vi "ABB Load-Save config.vi"(10 "confirm save":bool, 11 "Mode":enum16{"LOAD", "SAVE"}(ring)) -> ()   [LabVIEW 2017]
uses:
  ABB global.vi
panel:
  out "first row":string[](array[string])
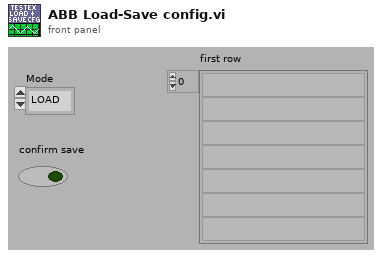
[diagram p1: front panel]
types:
  T1 = cluster{"First row[0]":string, "First row[1]":string, "First row[2]":string, "First row[3]":string, "First row[4]":string}
  T2 = cluster{"First row[0]":string, "First row[1]":string, "First row[2]":string, "First row[3]":string, "First row[4]":string, "First row[5]":string, "First row[6]":string, "First row[7]":string, "First row[8]":string}
  T3 = cluster{"Number Values":i32, "Tolerance":dbl, "Value (ratio) ":dbl[], "Hold time (sec)":dbl}
  T4 = cluster{"Thermal Stability (deg/hr)":dbl, "Reading interval (mins)":dbl}
  T5 = cluster{"Number Values":i32, "Tolerance ":dbl, "Value (ratio)":dbl[], "Hold time (sec)":dbl}
  T6 = cluster{"Simulate Norma":bool, "Norma 5000 Address":u8, "WebDaq IP Address":string, "Simulate cDAQ":bool}
  T7 = cluster{"temp. alloc":i32[], "category":i32[], "Category names":string[], "Category none names":string[]}
  T8 = cluster{"Number of Loads":i32, "Loads (%Rated)":dbl[]}
  T9 = cluster{"VT Primary":dbl, "VT Secondary":dbl, "CT  Primary":dbl, "CT Secondary":dbl, "Current Shunt":enum16{"Internal", "External"}, "Averaging interval":dbl}
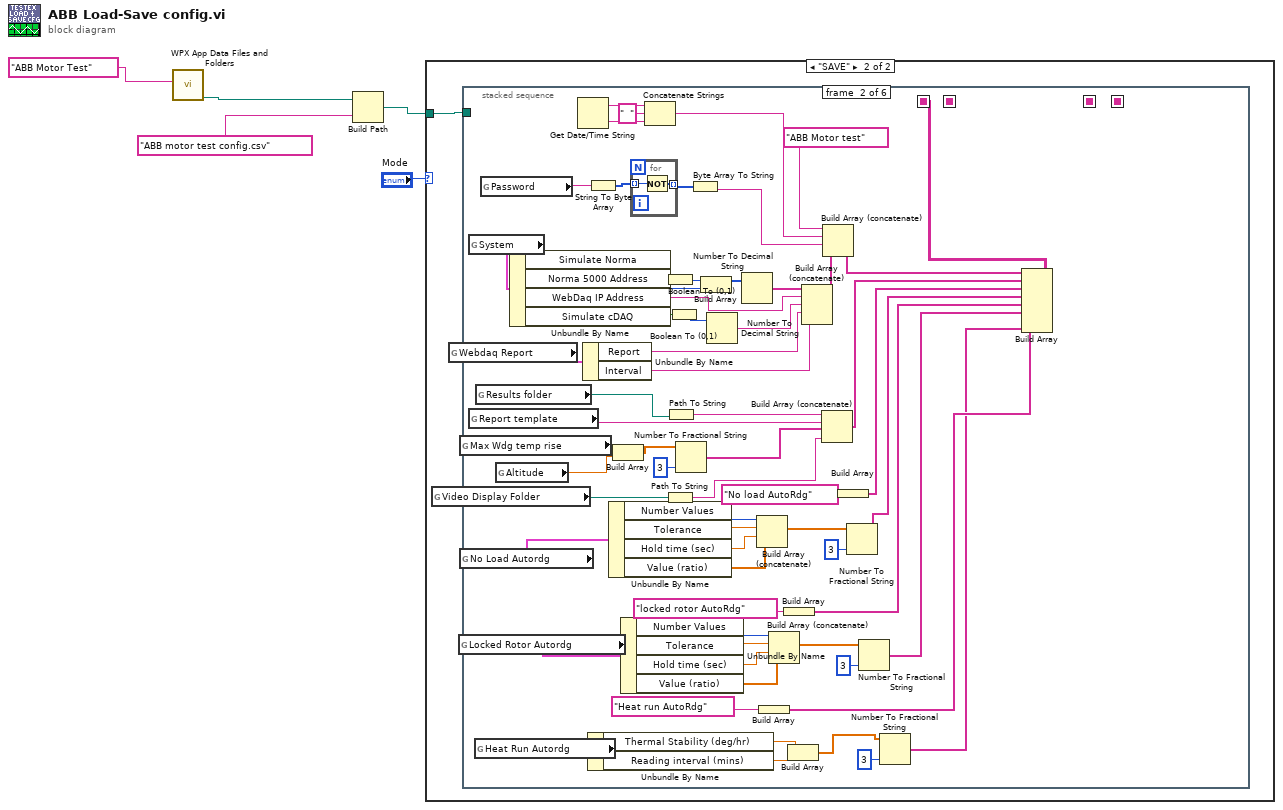
[diagram p0: block diagram]
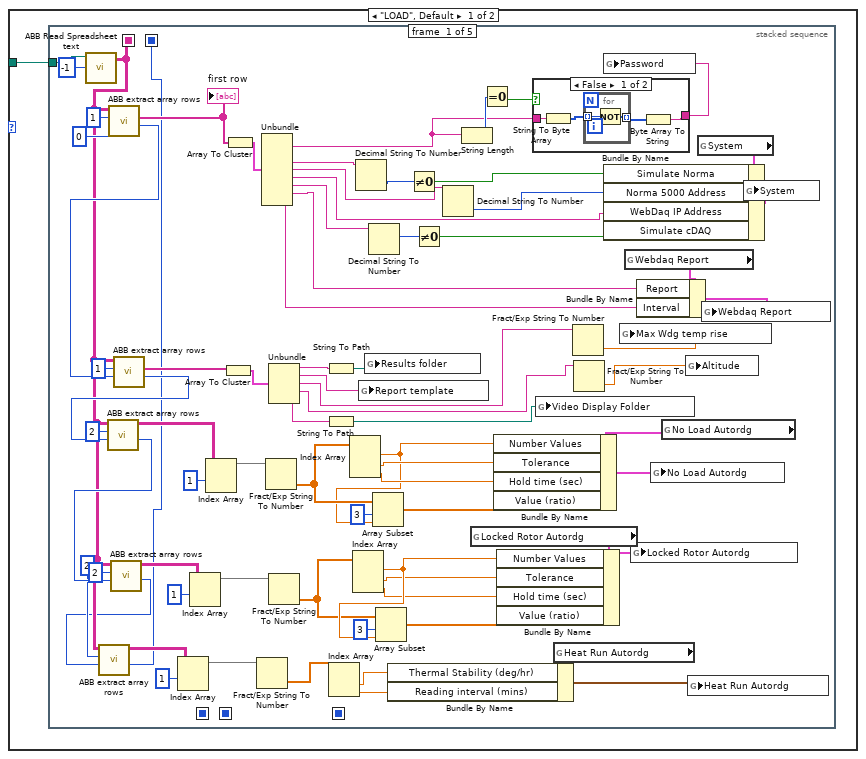
[diagram p2: hidden frame]
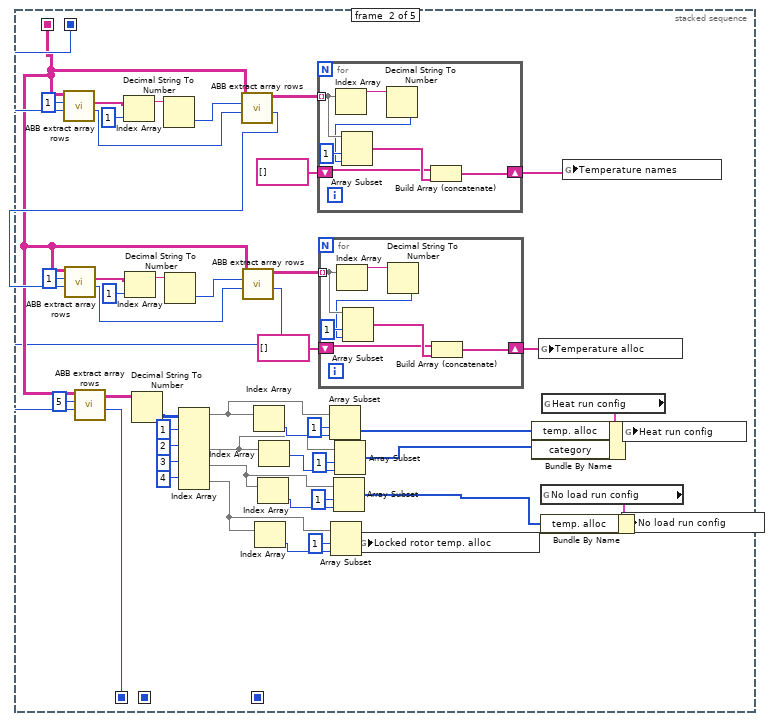
[diagram p4: hidden frame]
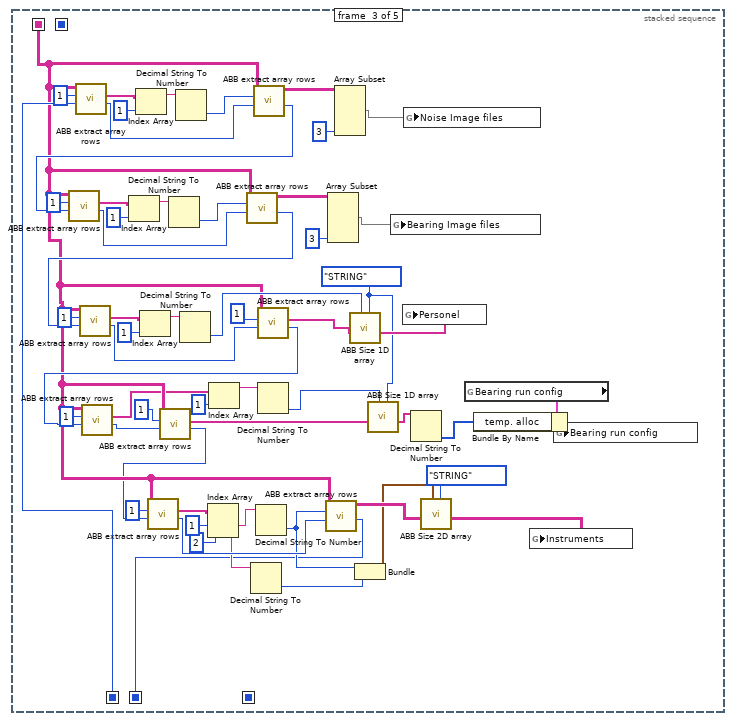
[diagram p5: hidden frame]
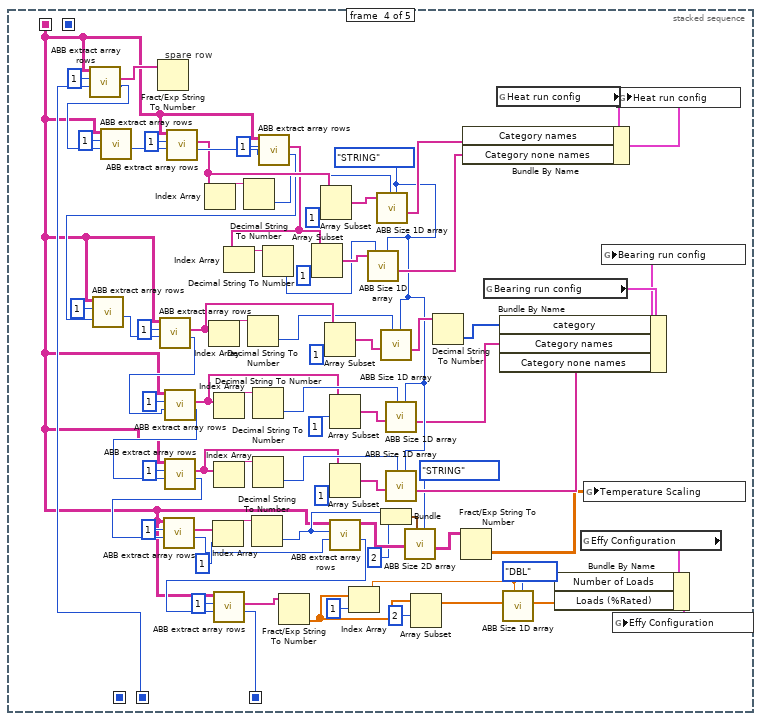
[diagram p6: hidden frame]
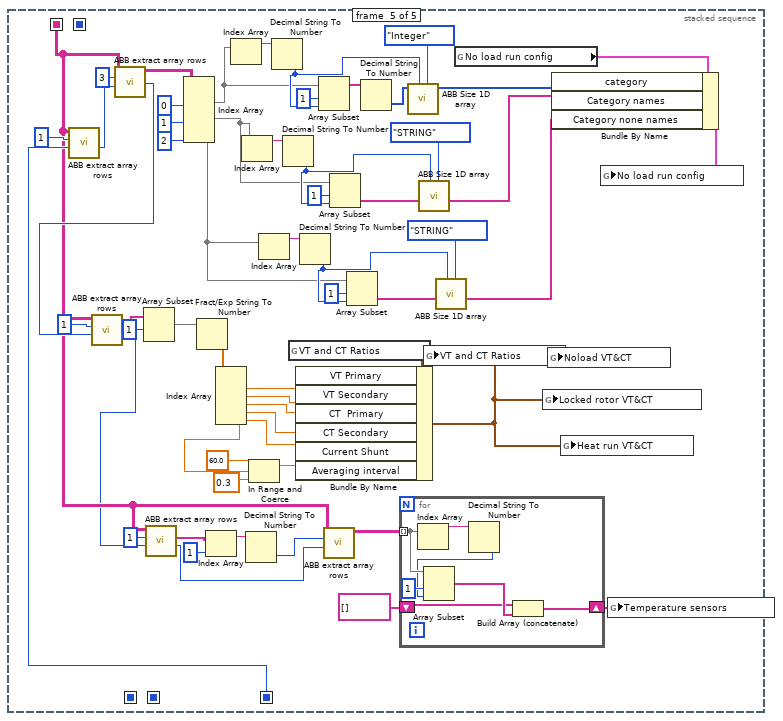
[diagram p7: hidden frame]
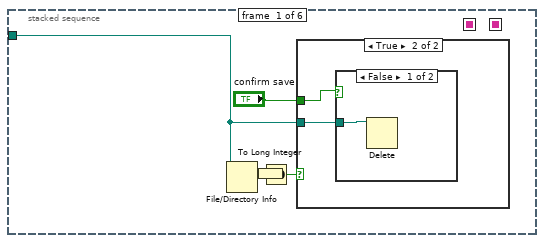
[diagram p8: hidden frame]
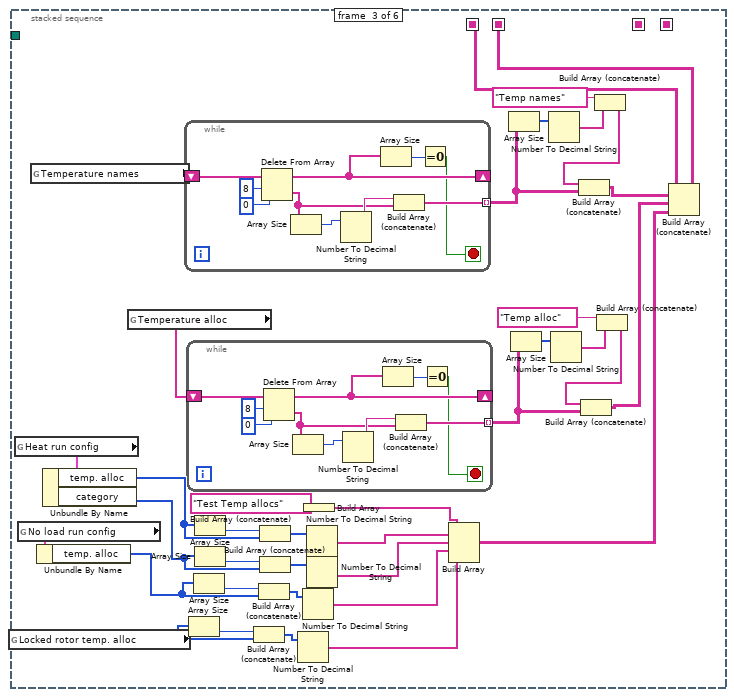
[diagram p11: hidden frame]
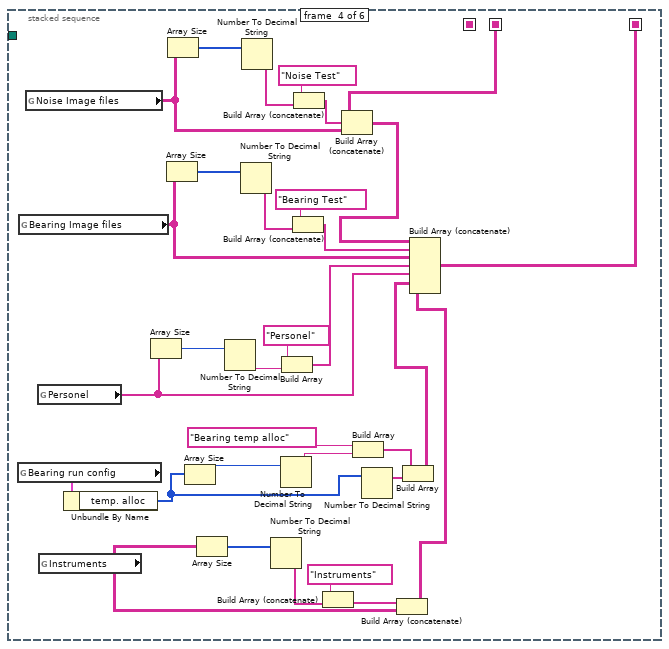
[diagram p12: hidden frame]
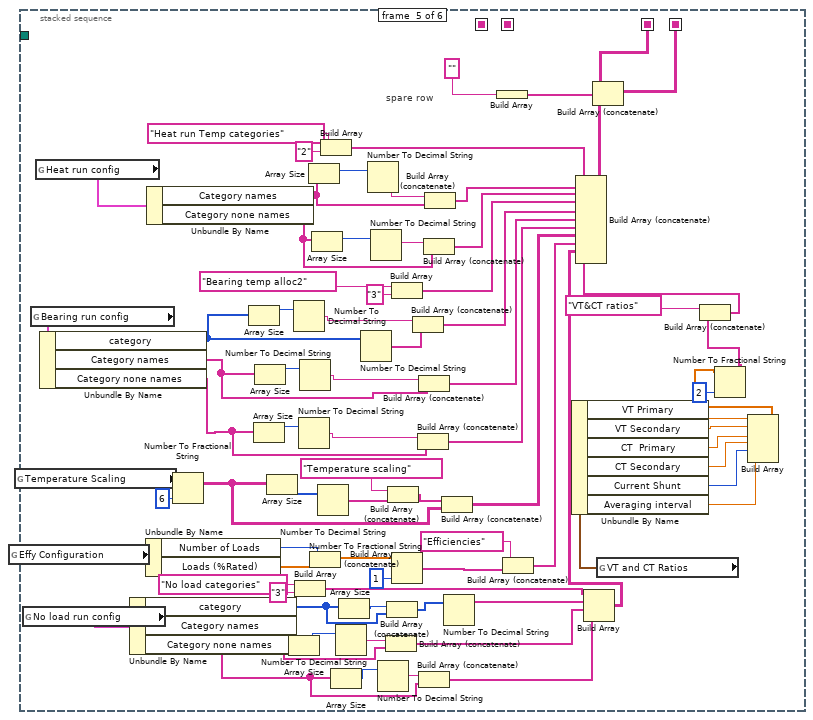
[diagram p13: hidden frame]
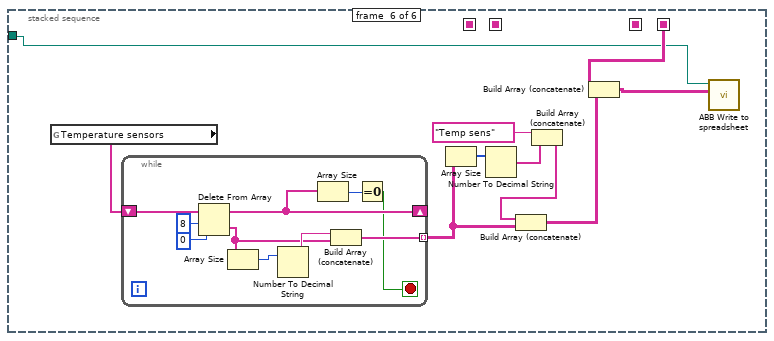
[diagram p14: hidden frame]
diagram:
  n1 = call "WPX App Data Files and Folders.vi"("ApplicationName"="ABB Motor Test") -> ("DataFolder"=w1:path)  [unwired: 7 in, 3 out]
  n2 = Build Path(base path=w1, name or relative path="ABB motor test config.csv") -> (appended path=w3:path)
  n3 = case shown="\"SAVE\"" "Mode" {
    tunnel: w3 -> [w6 w360]
    frame "LOAD", Default {
      n4 = stacked-sequence {
        seq-local: [w30 _ _ _ _] -> [_ w118 w162 w215 w295]
        seq-local: [w23 _ _ _ _] -> [_ w138 _ _ _]
        seq-local: [_ w103 _ _ _] -> [_ _ w207 _ _]
        seq-local: [_ _ w166 _ _] -> [_ _ _ w292 _]
        seq-local: [_ _ _ w214 _] -> [_ _ _ _ w351]
        tunnel: w6 -> [w77 _ _ _ _]
        frame #0 {
          n5 = call "ABB Read Spreadsheet text.vi"("number of rows (all:-1)"=-1, "file path (dialog if empty)"=w77) -> ("all rows"=w30:string[][])  [unwired: 5 in, 4 out]
          n6 = call "ABB extract array rows.vi"("Row offset"=0, "# rows"=1, "Input array"=w30) -> ("Next row"=w65:i32, "First row"=w74:string[])  [unwired: 6 in, 1 out]
          "first row" <- w74
          n7 = call "ABB extract array rows.vi"("Row offset"=w65, "# rows"=1, "Input array"=w30) -> ("Next row"=w59:i32, "First row"=w64:string[])  [unwired: 6 in, 1 out]
          n8 = call "ABB extract array rows.vi"("Row offset"=w59, "# rows"=2, "Input array"=w30) -> ("Next row"=w35:i32, "All rows"=w58:string[][])  [unwired: 6 in, 1 out]
          n9 = call "ABB extract array rows.vi"("Row offset"=w35, "# rows"=2, "Input array"=w30) -> ("Next row"=w29:i32, "All rows"=w37:string[][])  [unwired: 6 in, 1 out]
          n10 = call "ABB extract array rows.vi"("Row offset"=w29, "# rows"=2, "Input array"=w30) -> ("Next row"=w23:i32, "All rows"=w33:string[][])  [unwired: 6 in, 1 out]
          n11 = Index Array(array=w33, index (row)=1) -> (element=w31:string[])  [unwired: 1 in]
          n12 = Index Array(array=w37, index (row)=1) -> (element=w39:string[])  [unwired: 1 in]
          n13 = Index Array(array=w58, index (row)=1) -> (element=w56:string[])  [unwired: 1 in]
          n14 = Array To Cluster(array=w64) -> (cluster=w63:T1)
          n15 = Array To Cluster(array=w74) -> (cluster=w82:T2)
          n16 = Fract/Exp String To Number(string=w31) -> (number=w27:dbl[])  [unwired: 3 in, 1 out]
          n17 = Unbundle(w82) -> ("First row[2]"=w76:string, "First row[3]"=w72:string, "First row[4]"=w21:string, "First row[5]"=w20:string, "First row[6]"=w19:string, "First row[7]"=w9:string, "First row[8]"=w10:string)  [unwired: 2 out]
          n18 = Fract/Exp String To Number(string=w56) -> (number=w52:dbl[])  [unwired: 3 in, 1 out]
          n19 = Unbundle(w63) -> ("First row[0]"=w62:string, "First row[1]"=w22:string, "First row[2]"=w16:string, "First row[3]"=w15:string, "First row[4]"=w8:string)
          n20 = Fract/Exp String To Number(string=w39) -> (number=w43:dbl[])  [unwired: 3 in, 1 out]
          n21 = String To Path(string=w62) -> (path=w61:path)
          n22 = String To Path(string=w8) -> (path=w7:path)
          n23 = Index Array(array=w27) -> (element #1=w26:dbl, element #2=w25:dbl)  [unwired: 2 in]
          n24 = Index Array(array=w52) -> (element #1=w50:dbl, element #2=w54:dbl, element #3=w53:dbl)  [unwired: 3 in]
          n25 = Index Array(array=w43) -> (element #1=w45:dbl, element #2=w41:dbl, element #3=w42:dbl)  [unwired: 3 in]
          n26 = Decimal String To Number(string=w72) -> (number=w71:i32)  [unwired: 2 in, 1 out]
          n27 = global write "ABB global.vi" "Report template"(w22) -> ()
          n28 = global write "ABB global.vi" "Results folder"(w61) -> ()
          n29 = Decimal String To Number(string=w19) -> (number=w18:i32)  [unwired: 2 in, 1 out]
          n30 = Array Subset(array=w52, index=3, length=w50) -> (w49:dbl[])
          n31 = Array Subset(array=w43, index=3, length=w45) -> (w46:dbl[])
          n32 = Not Equal To 0?(x=w71) -> (x != 0?=w69:bool)
          n33 = Not Equal To 0?(x=w18) -> (x != 0?=w17:bool)
          n34 = Decimal String To Number(string=w21) -> (number=w68:i32)  [unwired: 2 in, 1 out]
          n35 = String Length(string=w76) -> (length=w81:i32)
          n36 = global read "ABB global.vi" "Locked Rotor Autordg"() -> (w40:T3)
          n37 = Equal To 0?(x=w81) -> (x = 0?=w80:bool)
          n38 = Bundle By Name(cluster=w40, "Number Values"=w45, "Tolerance"=w41, "Hold time (sec)"=w42, "Value (ratio)"=w46) -> (w47:T3)
          n39 = case shown="False" w80 {
            tunnel: w76 -> [w84 w89]
            tunnel: [w83 w89] -> w79
            frame False {
              n40 = String To Byte Array(string=w84) -> (unsigned byte array=w86:u8[])
              n41 = for {
                tunnel: w86 -> [w88] mode=indexing
                tunnel: [w87] -> w85 mode=indexing
                n42 = Not(x=w88) -> (.not. x?=w87:u8)
              }
              n43 = Byte Array To String(unsigned byte array=w85) -> (string=w83:string)
            }
            frame True {
            }
          }
          n44 = global write "ABB global.vi" "Video Display Folder"(w7) -> ()
          n45 = global read "ABB global.vi" "Heat Run Autordg"() -> (w28:T4)
          n46 = Bundle By Name(cluster=w28, "Thermal Stability (deg/hr)"=w26, "Reading interval (mins)"=w25) -> (w24:T4)
          n47 = Fract/Exp String To Number(string=w16) -> (number=w14:dbl)  [unwired: 3 in, 1 out]
          n48 = Fract/Exp String To Number(string=w15) -> (number=w13:dbl)  [unwired: 3 in, 1 out]
          n49 = global write "ABB global.vi" "Password"(w79) -> ()
          n50 = global write "ABB global.vi" "Max Wdg temp rise"(w14) -> ()
          n51 = global read "ABB global.vi" "Webdaq Report"() -> (w12:cluster{"Report":string, "Interval":string})
          n52 = global write "ABB global.vi" "Locked Rotor Autordg"(w47) -> ()
          n53 = Bundle By Name(cluster=w12, "Report"=w9, "Interval"=w10) -> (w11:cluster{"Report":string, "Interval":string})
          n54 = global read "ABB global.vi" "No Load Autordg"() -> (w55:T5)
          n55 = Bundle By Name(cluster=w55, "Number Values"=w50, "Tolerance"=w54, "Hold time (sec)"=w53, "Value (ratio)"=w49) -> (w48:T5)
          n56 = global write "ABB global.vi" "No Load Autordg"(w48) -> ()
          n57 = global write "ABB global.vi" "Altitude"(w13) -> ()
          n58 = global write "ABB global.vi" "Heat Run Autordg"(w24) -> ()
          n59 = global read "ABB global.vi" "System"() -> (w70:T6)
          n60 = Bundle By Name(cluster=w70, "Simulate Norma"=w69, "Norma 5000 Address"=w68, "WebDaq IP Address"=w20, "Simulate cDAQ"=w17) -> (w67:T6)
          n61 = global write "ABB global.vi" "Webdaq Report"(w11) -> ()
          n62 = global write "ABB global.vi" "System"(w67) -> ()
        }
        frame #1 {
          n63 = call "ABB extract array rows.vi"("Row offset"=w138, "# rows"=1, "Input array"=w118) -> ("Next row"=w134:i32, "First row"=w137:string[])  [unwired: 6 in, 1 out]
          n64 = Index Array(array=w137, index=1) -> (element=w135:string)
          n65 = Decimal String To Number(string=w135) -> (number=w133:i32)  [unwired: 2 in, 1 out]
          n66 = call "ABB extract array rows.vi"("Row offset"=w134, "# rows"=w133, "Input array"=w118) -> ("Next row"=w121:i32, "All rows"=w132:string[][])  [unwired: 6 in, 1 out]
          n67 = call "ABB extract array rows.vi"("Row offset"=w121, "# rows"=1, "Input array"=w118) -> ("Next row"=w126:i32, "First row"=w123:string[])  [unwired: 6 in, 1 out]
          n68 = Index Array(array=w123, index=1) -> (element=w125:string)
          n69 = Decimal String To Number(string=w125) -> (number=w127:i32)  [unwired: 2 in, 1 out]
          n70 = call "ABB extract array rows.vi"("Row offset"=w126, "# rows"=w127, "Input array"=w118) -> ("Next row"=w112:i32, "All rows"=w128:string[][])  [unwired: 6 in, 1 out]
          n71 = call "ABB extract array rows.vi"("Row offset"=w112, "# rows"=5, "Input array"=w118) -> ("Next row"=w103:i32, "All rows"=w117:string[][])  [unwired: 6 in, 1 out]
          n72 = Decimal String To Number(string=w117) -> (number=w116:i32[][])  [unwired: 2 in, 1 out]
          n73 = Index Array(array=w116, index (row) #1=1 ("index (row)"), index (row) #2=2 ("index (row)"), index (row) #3=3 ("index (row)"), index (row) #4=4 ("index (row)")) -> (element #1=w110:i32[], element #2=w97:i32[], element #3=w95:i32[], element #4=w94:i32[])  [unwired: 4 in]
          n74 = Index Array(array=w110) -> (element=w111:i32)  [unwired: 1 in]
          n75 = Index Array(array=w94) -> (element=w106:i32)  [unwired: 1 in]
          n76 = Index Array(array=w95) -> (element=w107:i32)  [unwired: 1 in]
          n77 = Index Array(array=w97) -> (element=w93:i32)  [unwired: 1 in]
          n78 = for {
            tunnel: w132 -> [w153] mode=indexing
            shift-right: [w147] -> w130
            shift-left: string[] [] -> [w148]
            n79 = Index Array(array=w153) -> (element=w151:string)  [unwired: 1 in]
            n80 = Decimal String To Number(string=w151) -> (number=w150:i32)  [unwired: 2 in, 1 out]
            n81 = Array Subset(array=w153, index=1, length=w150) -> (w149:string[])
            n82 = Build Array (concatenate)(w148, w149) -> (w147:string[])
          }
          n83 = for {
            tunnel: w128 -> [w146] mode=indexing
            shift-right: [w140] -> w120
            shift-left: string[] [] -> [w141]
            n84 = Index Array(array=w146) -> (element=w144:string)  [unwired: 1 in]
            n85 = Decimal String To Number(string=w144) -> (number=w143:i32)  [unwired: 2 in, 1 out]
            n86 = Array Subset(array=w146, index=1, length=w143) -> (w142:string[])
            n87 = Build Array (concatenate)(w141, w142) -> (w140:string[])
          }
          n88 = Array Subset(array=w110, index=1, length=w111) -> (w100:i32[])
          n89 = Array Subset(array=w94, index=1, length=w106) -> (w104:i32[])
          n90 = Array Subset(array=w95, index=1, length=w107) -> (w90:i32[])
          n91 = Array Subset(array=w97, index=1, length=w93) -> (w96:i32[])
          n92 = global write "ABB global.vi" "Locked rotor temp. alloc"(w104) -> ()
          n93 = global write "ABB global.vi" "Temperature alloc"(w120) -> ()
          n94 = global read "ABB global.vi" "No load run config"() -> (w91:T7)
          n95 = Bundle By Name(cluster=w91, "temp. alloc"=w90) -> (w92:T7)
          n96 = global read "ABB global.vi" "Heat run config"() -> (w102:T7)
          n97 = Bundle By Name(cluster=w102, "temp. alloc"=w100, "category"=w96) -> (w101:T7)
          n98 = global write "ABB global.vi" "Temperature names"(w130) -> ()
          n99 = global write "ABB global.vi" "No load run config"(w92) -> ()
          n100 = global write "ABB global.vi" "Heat run config"(w101) -> ()
        }
        frame #2 {
          w181 = enum16{"Integer", "DBL", "STRING", "BOOLEAN"}."STRING" ("Type")
          n101 = call "ABB extract array rows.vi"("Row offset"=w207, "# rows"=1, "Input array"=w162) -> ("Next row"=w212:i32, "First row"=w209:string[])  [unwired: 6 in, 1 out]
          n102 = Index Array(array=w209, index=1) -> (element=w211:string)
          n103 = Decimal String To Number(string=w211) -> (number=w213:i32)  [unwired: 2 in, 1 out]
          n104 = call "ABB extract array rows.vi"("Row offset"=w212, "# rows"=w213, "Input array"=w162) -> ("Next row"=w194:i32, "All rows"=w206:string[][])  [unwired: 6 in, 1 out]
          n105 = call "ABB extract array rows.vi"("Row offset"=w194, "# rows"=1, "Input array"=w162) -> ("Next row"=w196:i32, "First row"=w199:string[])  [unwired: 6 in, 1 out]
          n106 = Index Array(array=w199, index=1) -> (element=w197:string)
          n107 = Decimal String To Number(string=w197) -> (number=w195:i32)  [unwired: 2 in, 1 out]
          n108 = call "ABB extract array rows.vi"("Row offset"=w196, "# rows"=w195, "Input array"=w162) -> ("Next row"=w189:i32, "All rows"=w201:string[][])  [unwired: 6 in, 1 out]
          n109 = call "ABB extract array rows.vi"("Row offset"=w189, "# rows"=1, "Input array"=w162) -> ("Next row"=w185:i32, "First row"=w191:string[])  [unwired: 6 in, 1 out]
          n110 = Index Array(array=w191, index=1) -> (element=w193:string)
          n111 = Decimal String To Number(string=w193) -> (number=w182:i32)  [unwired: 2 in, 1 out]
          n112 = call "ABB extract array rows.vi"("Row offset"=w185, "# rows"=1, "Input array"=w162) -> ("Next row"=w187:i32, "First row"=w184:string[])  [unwired: 6 in, 1 out]
          n113 = call "ABB extract array rows.vi"("Row offset"=w187, "# rows"=1, "Input array"=w162) -> ("Next row"=w161:i32, "First row"=w157:string[])  [unwired: 6 in, 1 out]
          n114 = call "ABB extract array rows.vi"("Row offset"=w161, "# rows"=1, "Input array"=w162) -> ("Next row"=w160:i32, "First row"=w158:string[])  [unwired: 6 in, 1 out]
          n115 = call "ABB extract array rows.vi"("Row offset"=w160, "# rows"=1, "Input array"=w162) -> ("Next row"=w179:i32, "First row"=w176:string[])  [unwired: 6 in, 1 out]
          n116 = Index Array(array=w176, index #1=1 ("index"), index #2=2 ("index")) -> (element #1=w178:string, element #2=w171:string)
          n117 = Index Array(array=w157, index=1) -> (element=w155:string)
          n118 = Decimal String To Number(string=w171) -> (number=w169:i32)  [unwired: 2 in, 1 out]
          n119 = Decimal String To Number(string=w178) -> (number=w170:i32)  [unwired: 2 in, 1 out]
          n120 = Decimal String To Number(string=w155) -> (number=w154:i32)  [unwired: 2 in, 1 out]
          n121 = call "ABB extract array rows.vi"("Row offset"=w179, "# rows"=w170, "Input array"=w162) -> ("Next row"=w166:i32, "All rows"=w174:string[][])  [unwired: 6 in, 1 out]
          n122 = Array Subset(array=w201, length (col)=3 ("length")) -> (w203:string[][])  [unwired: 3 in]
          n123 = Array Subset(array=w206, length (col)=3 ("length")) -> (w204:string[][])  [unwired: 3 in]
          n124 = call "ABB Size 1D array.vi"("Type"=w181, "Size"=w182, "String Array in"=w184) -> ("String Array out"=w183:string[])  [unwired: 5 in, 3 out]
          n125 = Bundle(w170, w169) -> (w168:cluster{i32, i32})  [unwired: 1 in]
          n126 = call "ABB Size 1D array.vi"("Type"=w181, "Size"=w154, "String Array in"=w158) -> ("String Array out"=w180:string[])  [unwired: 5 in, 3 out]
          n127 = global write "ABB global.vi" "Bearing Image files"(w203) -> ()
          n128 = global write "ABB global.vi" "Personel"(w183) -> ()
          n129 = global write "ABB global.vi" "Noise Image files"(w204) -> ()
          n130 = Decimal String To Number(string=w180) -> (number=w164:i32[])  [unwired: 2 in, 1 out]
          n131 = call "ABB Size 2D array.vi"("Type"=enum16{"Integer", "DBL", "STRING", "BOOLEAN"}."STRING", "Size"=w168, "String Array in"=w174) -> ("String Array out"=w167:string[][])  [unwired: 5 in, 3 out]
          n132 = global read "ABB global.vi" "Bearing run config"() -> (w165:T7)
          n133 = Bundle By Name(cluster=w165, "temp. alloc"=w164) -> (w163:T7)
          n134 = global write "ABB global.vi" "Instruments"(w167) -> ()
          n135 = global write "ABB global.vi" "Bearing run config"(w163) -> ()
        }
        frame #3 {
          w243 = enum16{"Integer", "DBL", "STRING", "BOOLEAN"}."STRING" ("Type")
          # "spare row"
          n136 = call "ABB extract array rows.vi"("Row offset"=w292, "# rows"=1, "Input array"=w215) -> ("Next row"=w285:i32, "First row"=w291:string[])  [unwired: 6 in, 1 out]
          n137 = call "ABB extract array rows.vi"("Row offset"=w285, "# rows"=1, "Input array"=w215) -> ("Next row"=w284:i32)  [unwired: 6 in, 2 out]
          n138 = Fract/Exp String To Number(string=w291) -> ()  [unwired: 3 in, 2 out]
          n139 = call "ABB extract array rows.vi"("Row offset"=w284, "# rows"=1, "Input array"=w215) -> ("Next row"=w283:i32, "First row"=w281:string[])  [unwired: 6 in, 1 out]
          n140 = Index Array(array=w281) -> (element=w282:string)  [unwired: 1 in]
          n141 = Decimal String To Number(string=w282) -> (number=w277:i32)  [unwired: 2 in, 1 out]
          n142 = call "ABB extract array rows.vi"("Row offset"=w283, "# rows"=1, "Input array"=w215) -> ("Next row"=w265:i32, "First row"=w273:string[])  [unwired: 6 in, 1 out]
          n143 = call "ABB extract array rows.vi"("Row offset"=w265, "# rows"=1, "Input array"=w215) -> ("Next row"=w268:i32)  [unwired: 6 in, 2 out]
          n144 = call "ABB extract array rows.vi"("Row offset"=w268, "# rows"=1, "Input array"=w215) -> ("Next row"=w247:i32, "First row"=w262:string[])  [unwired: 6 in, 1 out]
          n145 = call "ABB extract array rows.vi"("Row offset"=w247, "# rows"=1, "Input array"=w215) -> ("Next row"=w246:i32, "First row"=w245:string[])  [unwired: 6 in, 1 out]
          n146 = call "ABB extract array rows.vi"("Row offset"=w246, "# rows"=1, "Input array"=w215) -> ("Next row"=w237:i32, "First row"=w244:string[])  [unwired: 6 in, 1 out]
          n147 = call "ABB extract array rows.vi"("Row offset"=w237, "# rows"=1, "Input array"=w215) -> ("Next row"=w235:i32, "First row"=w240:string[])  [unwired: 6 in, 1 out]
          n148 = Index Array(array=w262) -> (element=w260:string)  [unwired: 1 in]
          n149 = Index Array(array=w240, index=1) -> (element=w239:string)
          n150 = Index Array(array=w245) -> (element=w257:string)  [unwired: 1 in]
          n151 = Index Array(array=w244) -> (element=w248:string)  [unwired: 1 in]
          n152 = Index Array(array=w273) -> (element=w274:string)  [unwired: 1 in]
          n153 = Decimal String To Number(string=w260) -> (number=w261:i32)  [unwired: 2 in, 1 out]
          n154 = Decimal String To Number(string=w239) -> (number=w232:i32)  [unwired: 2 in, 1 out]
          n155 = Decimal String To Number(string=w257) -> (number=w256:i32)  [unwired: 2 in, 1 out]
          n156 = Decimal String To Number(string=w248) -> (number=w249:i32)  [unwired: 2 in, 1 out]
          n157 = Decimal String To Number(string=w274) -> (number=w272:i32)  [unwired: 2 in, 1 out]
          n158 = Array Subset(array=w273, index=1) -> (w276:string[])  [unwired: 1 in]
          n159 = Array Subset(array=w281, index=1) -> (w279:string[])  [unwired: 1 in]
          n160 = Array Subset(array=w262, index=1) -> (w264:string[])  [unwired: 1 in]
          n161 = Array Subset(array=w245, index=1) -> (w254:string[])  [unwired: 1 in]
          n162 = Array Subset(array=w244, index=1) -> (w251:string[])  [unwired: 1 in]
          n163 = call "ABB extract array rows.vi"("Row offset"=w235, "# rows"=w232, "Input array"=w215) -> ("Next row"=w226:i32, "All rows"=w234:string[][])  [unwired: 6 in, 1 out]
          n164 = call "ABB extract array rows.vi"("Row offset"=w226, "# rows"=1, "Input array"=w215) -> ("Next row"=w214:i32, "First row"=w225:string[])  [unwired: 6 in, 1 out]
          n165 = Fract/Exp String To Number(string=w225) -> (number=w223:dbl[])  [unwired: 3 in, 1 out]
          n166 = Index Array(array=w223, index=1) -> (element=w219:dbl)
          n167 = call "ABB Size 1D array.vi"("Type"=w243, "Size"=w272, "String Array in"=w276) -> ("String Array out"=w271:string[])  [unwired: 5 in, 3 out]
          n168 = call "ABB Size 1D array.vi"("Type"=w243, "Size"=w277, "String Array in"=w279) -> ("String Array out"=w278:string[])  [unwired: 5 in, 3 out]
          n169 = call "ABB Size 1D array.vi"("Type"=w243, "Size"=w261, "String Array in"=w264) -> ("String Array out"=w259:string[])  [unwired: 5 in, 3 out]
          n170 = Bundle(w232, 2) -> (w230:cluster{i32, i32})  [unwired: 1 in]
          n171 = call "ABB Size 1D array.vi"("Type"=w243, "Size"=w256, "String Array in"=w254) -> ("String Array out"=w241:string[])  [unwired: 5 in, 3 out]
          n172 = call "ABB Size 1D array.vi"("Type"=w243, "Size"=w249, "String Array in"=w251) -> ("String Array out"=w242:string[])  [unwired: 5 in, 3 out]
          n173 = call "ABB Size 2D array.vi"("Type"=enum16{"Integer", "DBL", "STRING", "BOOLEAN"}."STRING", "Size"=w230, "String Array in"=w234) -> ("String Array out"=w229:string[][])  [unwired: 5 in, 3 out]
          n174 = Array Subset(array=w223, index=2) -> (w220:dbl[])  [unwired: 1 in]
          n175 = Decimal String To Number(string=w259) -> (number=w258:i32[])  [unwired: 2 in, 1 out]
          n176 = Fract/Exp String To Number(string=w229) -> (number=w228:dbl[][])  [unwired: 3 in, 1 out]
          n177 = global read "ABB global.vi" "Bearing run config"() -> (w270:T7)
          n178 = global read "ABB global.vi" "Heat run config"() -> (w290:T7)
          n179 = Bundle By Name(cluster=w290, "Category names"=w278, "Category none names"=w271) -> (w289:T7)
          n180 = Bundle By Name(cluster=w270, "category"=w258, "Category names"=w241, "Category none names"=w242) -> (w269:T7)
          n181 = call "ABB Size 1D array.vi"("Type"=enum16{"Integer", "DBL", "STRING", "BOOLEAN"}."DBL", "Size"=w219, "DBL Array In"=w220) -> ("DBL Array out"=w216:dbl[])  [unwired: 5 in, 3 out]
          n182 = global read "ABB global.vi" "Effy Configuration"() -> (w221:T8)
          n183 = Bundle By Name(cluster=w221, "Number of Loads"=w219, "Loads (%Rated)"=w216) -> (w217:T8)
          n184 = global write "ABB global.vi" "Temperature Scaling"(w228) -> ()
          n185 = global write "ABB global.vi" "Bearing run config"(w269) -> ()
          n186 = global write "ABB global.vi" "Effy Configuration"(w217) -> ()
          n187 = global write "ABB global.vi" "Heat run config"(w289) -> ()
        }
        frame #4 {
          n188 = call "ABB extract array rows.vi"("Row offset"=w351, "# rows"=1, "Input array"=w295) -> ("Next row"=w349:i32)  [unwired: 6 in, 2 out]
          n189 = call "ABB extract array rows.vi"("Row offset"=w349, "# rows"=3, "Input array"=w295) -> ("Next row"=w319:i32, "All rows"=w339:string[][])  [unwired: 6 in, 1 out]
          n190 = call "ABB extract array rows.vi"("Row offset"=w319, "# rows"=1, "Input array"=w295) -> ("Next row"=w294:i32, "First row"=w311:string[])  [unwired: 6 in, 1 out]
          n191 = Array Subset(array=w311, index=1) -> (w312:string[])  [unwired: 1 in]
          n192 = call "ABB extract array rows.vi"("Row offset"=w294, "# rows"=1, "Input array"=w295) -> ("Next row"=w301:i32, "First row"=w298:string[])  [unwired: 6 in, 1 out]
          n193 = Index Array(array=w339, index (row) #1=0 ("index (row)"), index (row) #2=1 ("index (row)"), index (row) #3=2 ("index (row)")) -> (element #1=w338:string[], element #2=w326:string[], element #3=w321:string[])  [unwired: 3 in]
          n194 = Fract/Exp String To Number(string=w312) -> (number=w317:dbl[])  [unwired: 3 in, 1 out]
          n195 = Index Array(array=w298, index=1) -> (element=w300:string)
          n196 = Index Array(array=w317) -> (element #1=w316:dbl, element #2=w315:dbl, element #3=w314:dbl, element #4=w313:dbl, element #5=w308:dbl)  [unwired: 5 in]
          n197 = Index Array(array=w338) -> (element=w348:string)  [unwired: 1 in]
          n198 = Index Array(array=w326) -> (element=w331:string)  [unwired: 1 in]
          n199 = Decimal String To Number(string=w300) -> (number=w302:i32)  [unwired: 2 in, 1 out]
          n200 = In Range and Coerce(upper limit=60.0, x=w308, lower limit=0.3) -> (coerced(x)=w307:dbl)  [unwired: 1 out]
          n201 = Index Array(array=w321) -> (element=w330:string)  [unwired: 1 in]
          n202 = Decimal String To Number(string=w348) -> (number=w340:i32)  [unwired: 2 in, 1 out]
          n203 = Decimal String To Number(string=w331) -> (number=w334:i32)  [unwired: 2 in, 1 out]
          n204 = global read "ABB global.vi" "VT and CT Ratios"() -> (w318:T9)
          n205 = Bundle By Name(cluster=w318, "VT Primary"=w316, "VT Secondary"=w315, "CT  Primary"=w314, "CT Secondary"=w313, "Current Shunt"=w308, "Averaging interval"=w307) -> (w305:T9)
          n206 = Decimal String To Number(string=w330) -> (number=w327:i32)  [unwired: 2 in, 1 out]
          n207 = Array Subset(array=w338, index=1, length=w340) -> (w344:string[])
          n208 = call "ABB extract array rows.vi"("Row offset"=w301, "# rows"=w302, "Input array"=w295) -> ("All rows"=w303:string[][])  [unwired: 6 in, 2 out]
          n209 = Array Subset(array=w326, index=1, length=w334) -> (w325:string[])
          n210 = Array Subset(array=w321, index=1, length=w327) -> (w323:string[])
          n211 = Decimal String To Number(string=w344) -> (number=w343:i32[])  [unwired: 2 in, 1 out]
          n212 = for {
            tunnel: w303 -> [w359] mode=indexing
            shift-right: [w353] -> w296
            shift-left: string[] [] -> [w354]
            n213 = Index Array(array=w359) -> (element=w357:string)  [unwired: 1 in]
            n214 = Decimal String To Number(string=w357) -> (number=w356:i32)  [unwired: 2 in, 1 out]
            n215 = Array Subset(array=w359, index=1, length=w356) -> (w355:string[])
            n216 = Build Array (concatenate)(w354, w355) -> (w353:string[])
          }
          n217 = call "ABB Size 1D array.vi"("Type"=enum16{"Integer", "DBL", "STRING", "BOOLEAN"}."Integer", "Size"=w340, "Integer Array In"=w343) -> ("Integer Array Out"=w342:i32[])  [unwired: 5 in, 3 out]
          n218 = call "ABB Size 1D array.vi"("Type"=enum16{"Integer", "DBL", "STRING", "BOOLEAN"}."STRING", "Size"=w334, "String Array in"=w325) -> ("String Array out"=w324:string[])  [unwired: 5 in, 3 out]
          n219 = global write "ABB global.vi" "VT and CT Ratios"(w305) -> ()
          n220 = call "ABB Size 1D array.vi"("Type"=enum16{"Integer", "DBL", "STRING", "BOOLEAN"}."STRING", "Size"=w327, "String Array in"=w323) -> ("String Array out"=w322:string[])  [unwired: 5 in, 3 out]
          n221 = global read "ABB global.vi" "No load run config"() -> (w346:T7)
          n222 = global write "ABB global.vi" "Locked rotor VT&CT"(w305) -> ()
          n223 = global write "ABB global.vi" "Noload VT&CT"(w305) -> ()
          n224 = Bundle By Name(cluster=w346, "category"=w342, "Category names"=w324, "Category none names"=w322) -> (w345:T7)
          n225 = global write "ABB global.vi" "Heat run VT&CT"(w305) -> ()
          n226 = global write "ABB global.vi" "No load run config"(w345) -> ()
          n227 = global write "ABB global.vi" "Temperature sensors"(w296) -> ()
        }
      }
    }
    frame "SAVE" {
      n228 = stacked-sequence {
        seq-local: [_ w422 _ _ _ _] -> [_ _ w465 _ _ _]
        seq-local: [_ _ w463 _ _ _] -> [_ _ _ w518 _ _]
        seq-local: [_ _ _ w494 _ _] -> [_ _ _ _ w602 _]
        seq-local: [_ _ _ _ w524 _] -> [_ _ _ _ _ w612]
        tunnel: w360 -> [w362 _ _ _ _ w604]
        frame #0 {
          n229 = File/Directory Info(path=w362) -> (size=w361:i64)  [unwired: 1 in, 6 out]
          n230 = To Long Integer(number=w361) -> (32bit integer=w365:i32)
          n231 = Not Equal To 0?(x=w365) -> (x != 0?=w364:bool)
          n232 = case shown="True" w364 {
            tunnel: "confirm save" -> [_ w367]
            tunnel: w362 -> [_ w366]
            frame False {
            }
            frame True {
              n233 = case shown="False" w367 {
                tunnel: w366 -> [w368 _]
                frame False {
                  n234 = Delete(path (use dialog)=w368) -> ()  [unwired: 4 in, 3 out]
                }
                frame True {
                }
              }
            }
          }
        }
        frame #1 {
          n235 = global read "ABB global.vi" "Video Display Folder"() -> (w370:path)
          n236 = global read "ABB global.vi" "Webdaq Report"() -> (w373:cluster{"Report":string, "Interval":string})
          n237 = global read "ABB global.vi" "Locked Rotor Autordg"() -> (w395:T3)
          n238 = global read "ABB global.vi" "Max Wdg temp rise"() -> (w378:dbl)
          n239 = global read "ABB global.vi" "No Load Autordg"() -> (w412:T5)
          n240 = global read "ABB global.vi" "System"() -> (w421:T6)
          n241 = global read "ABB global.vi" "Report template"() -> (w384:string)
          n242 = global read "ABB global.vi" "Heat Run Autordg"() -> (w392:T4)
          n243 = global read "ABB global.vi" "Results folder"() -> (w415:path)
          n244 = global read "ABB global.vi" "Password"() -> (w430:string)
          n245 = global read "ABB global.vi" "Altitude"() -> (w377:dbl)
          n246 = Unbundle By Name(w421) -> ("Simulate Norma"=w420:bool, "Norma 5000 Address"=w418:u8, "WebDaq IP Address"=w382:string, "Simulate cDAQ"=w381:bool)
          n247 = Get Date/Time String() -> (date string=w428:string, time string=w427:string)  [unwired: 3 in]
          n248 = Unbundle By Name(w373) -> ("Report"=w372:string, "Interval"=w371:string)
          n249 = String To Byte Array(string=w430) -> (unsigned byte array=w432:u8[])
          n250 = Unbundle By Name(w392) -> ("Thermal Stability (deg/hr)"=w390:dbl, "Reading interval (mins)"=w389:dbl)
          n251 = Unbundle By Name(w412) -> ("Number Values"=w411:i32, "Tolerance"=w410:dbl, "Hold time (sec)"=w407:dbl, "Value (ratio)"=w406:dbl[])
          n252 = Build Array(w378, w377) -> (w376:dbl[])
          n253 = Unbundle By Name(w395) -> ("Number Values"=w396:i32, "Tolerance"=w397:dbl, "Hold time (sec)"=w400:dbl, "Value (ratio)"=w401:dbl[])
          n254 = for {
            tunnel: w432 -> [w434] mode=indexing
            tunnel: [w433] -> w431 mode=indexing
            n255 = Not(x=w434) -> (.not. x?=w433:u8)
          }
          n256 = Concatenate Strings(w428, "  " ("string"), w427) -> (w425:string)
          n257 = Boolean To (0,1)(Boolean=w420) -> (0, 1=w419:i16)
          n258 = Path To String(path=w370) -> (string=w369:string)
          n259 = Path To String(path=w415) -> (string=w413:string)
          n260 = Boolean To (0,1)(Boolean=w381) -> (0, 1=w380:i16)
          n261 = Number To Fractional String(number=w376, precision (6)=i16 3) -> (F-format string=w374:string[])  [unwired: 2 in]
          n262 = Byte Array To String(unsigned byte array=w431) -> (string=w429:string)
          n263 = Build Array(w419, w418) -> (w417:i16[])
          n264 = Number To Decimal String(number=w380) -> (decimal integer string=w379:string)  [unwired: 1 in]
          n265 = Number To Decimal String(number=w417) -> (decimal integer string=w416:string[])  [unwired: 1 in]
          n266 = Build Array (concatenate)(w411, w410, w407, w406) -> (w409:dbl[])
          n267 = Build Array("Heat run AutoRdg") -> (w388:string[])
          n268 = Build Array (concatenate)(w396, w397, w400, w401) -> (w398:dbl[])
          n269 = Build Array("locked rotor AutoRdg") -> (w394:string[])
          n270 = Build Array(w390, w389) -> (w386:dbl[])
          n271 = Build Array (concatenate)(w416, w382, w379, w372, w371) -> (w383:string[])
          n272 = Build Array (concatenate)(w413, w384, w374, w369) -> (w414:string[])
          n273 = Build Array (concatenate)("ABB Motor test", w425, w429, w383) -> (w423:string[])
          n274 = Build Array("No load AutoRdg") -> (w404:string[])
          n275 = Number To Fractional String(number=w409, precision (6)=i16 3) -> (F-format string=w403:string[])  [unwired: 2 in]
          n276 = Number To Fractional String(number=w398, precision (6)=i16 3) -> (F-format string=w393:string[])  [unwired: 2 in]
          n277 = Number To Fractional String(number=w386, precision (6)=i16 3) -> (F-format string=w385:string[])  [unwired: 2 in]
          n278 = Build Array(w423, w414, w404, w403, w394, w393, w388, w385) -> (w422:string[][])
        }
        frame #2 {
          n279 = global read "ABB global.vi" "Locked rotor temp. alloc"() -> (w446:i32[])
          n280 = global read "ABB global.vi" "Heat run config"() -> (w442:T7)
          n281 = global read "ABB global.vi" "No load run config"() -> (w436:T7)
          n282 = global read "ABB global.vi" "Temperature names"() -> (w471:string[])
          n283 = Unbundle By Name(w436) -> ("temp. alloc"=w435:i32[])
          n284 = Unbundle By Name(w442) -> ("temp. alloc"=w441:i32[], "category"=w438:i32[])
          n285 = global read "ABB global.vi" "Temperature alloc"() -> (w457:string[])
          n286 = while {
            shift-right: [w485] -> _
            shift-left: w471 -> [w491]
            tunnel: [w486] -> w466 mode=indexing
            stop <- w483 stop-if-true
            n287 = Delete From Array(array=w491, length=8, index=0) -> (deleted portion=w487:string[], array with subset deleted=w485:string[])
            n288 = Array Size(array=w487) -> (size(s)=w489:i32)
            n289 = Number To Decimal String(number=w489) -> (decimal integer string=w488:string)  [unwired: 1 in]
            n290 = Array Size(array=w485) -> (size(s)=w484:i32)
            n291 = Build Array (concatenate)(w488, w487) -> (w486:string[])
            n292 = Equal To 0?(x=w484) -> (x = 0?=w483:bool)
          }
          n293 = while {
            shift-right: [w475] -> _
            shift-left: w457 -> [w481]
            tunnel: [w476] -> w462 mode=indexing
            stop <- w473 stop-if-true
            n294 = Delete From Array(array=w481, length=8, index=0) -> (deleted portion=w477:string[], array with subset deleted=w475:string[])
            n295 = Array Size(array=w477) -> (size(s)=w479:i32)
            n296 = Number To Decimal String(number=w479) -> (decimal integer string=w478:string)  [unwired: 1 in]
            n297 = Array Size(array=w475) -> (size(s)=w474:i32)
            n298 = Build Array (concatenate)(w478, w477) -> (w476:string[])
            n299 = Equal To 0?(x=w474) -> (x = 0?=w473:bool)
          }
          n300 = Array Size(array=w446) -> (size(s)=w447:i32)
          n301 = Array Size(array=w435) -> (size(s)=w450:i32)
          n302 = Array Size(array=w441) -> (size(s)=w451:i32)
          n303 = Array Size(array=w438) -> (size(s)=w440:i32)
          n304 = Build Array (concatenate)(w447, w446) -> (w448:i32[])
          n305 = Build Array (concatenate)(w450, w435) -> (w449:i32[])
          n306 = Build Array (concatenate)(w451, w441) -> (w452:i32[])
          n307 = Build Array (concatenate)(w440, w438) -> (w439:i32[])
          n308 = Number To Decimal String(number=w448) -> (decimal integer string=w444:string[])  [unwired: 1 in]
          n309 = Number To Decimal String(number=w449) -> (decimal integer string=w445:string[])  [unwired: 1 in]
          n310 = Build Array("Test Temp allocs") -> (w454:string[])
          n311 = Number To Decimal String(number=w452) -> (decimal integer string=w453:string[])  [unwired: 1 in]
          n312 = Number To Decimal String(number=w439) -> (decimal integer string=w437:string[])  [unwired: 1 in]
          n313 = Build Array(w454, w453, w437, w445, w444) -> (w443:string[][])
          n314 = Array Size(array=w466) -> (size(s)=w470:i32[])
          n315 = Array Size(array=w462) -> (size(s)=w458:i32[])
          n316 = Number To Decimal String(number=w470) -> (decimal integer string=w468:string[])  [unwired: 1 in]
          n317 = Number To Decimal String(number=w458) -> (decimal integer string=w460:string[])  [unwired: 1 in]
          n318 = Build Array (concatenate)("Temp names", w468) -> (w467:string[])
          n319 = Build Array (concatenate)(w467, w466) -> (w464:string[][])
          n320 = Build Array (concatenate)("Temp alloc", w460) -> (w461:string[])
          n321 = Build Array (concatenate)(w461, w462) -> (w456:string[][])
          n322 = Build Array (concatenate)(w465, w464, w456, w443) -> (w463:string[][])
        }
        frame #3 {
          n323 = global read "ABB global.vi" "Bearing run config"() -> (w493:T7)
          n324 = global read "ABB global.vi" "Bearing Image files"() -> (w517:string[][])
          n325 = global read "ABB global.vi" "Noise Image files"() -> (w519:string[][])
          n326 = global read "ABB global.vi" "Personel"() -> (w507:string[])
          n327 = global read "ABB global.vi" "Instruments"() -> (w496:string[][])
          n328 = Unbundle By Name(w493) -> ("temp. alloc"=w492:i32[])
          n329 = Array Size(array=w507) -> (size(s)=w511:i32)
          n330 = Array Size(array=w517) -> (size(s)=w513:i32[])
          n331 = Array Size(array=w519) -> (size(s)=w523:i32[])
          n332 = Array Size(array=w492) -> (size(s)=w503:i32)
          n333 = Array Size(array=w496) -> (size(s)=w500:i32[])
          n334 = Number To Decimal String(number=w511) -> (decimal integer string=w510:string)  [unwired: 1 in]
          n335 = Number To Decimal String(number=w513) -> (decimal integer string=w514:string[])  [unwired: 1 in]
          n336 = Number To Decimal String(number=w523) -> (decimal integer string=w522:string[])  [unwired: 1 in]
          n337 = Number To Decimal String(number=w500) -> (decimal integer string=w499:string[])  [unwired: 1 in]
          n338 = Number To Decimal String(number=w503) -> (decimal integer string=w505:string)  [unwired: 1 in]
          n339 = Build Array("Personel", w510) -> (w508:string[])
          n340 = Build Array (concatenate)("Bearing Test", w514) -> (w516:string[])
          n341 = Build Array (concatenate)("Noise Test", w522) -> (w520:string[])
          n342 = Build Array (concatenate)("Instruments", w499) -> (w497:string[])
          n343 = Build Array (concatenate)(w518, w520, w519) -> (w512:string[][])
          n344 = Build Array("Bearing temp alloc", w505) -> (w504:string[])
          n345 = Number To Decimal String(number=w492) -> (decimal integer string=w502:string[])  [unwired: 1 in]
          n346 = Build Array (concatenate)(w497, w496) -> (w495:string[][])
          n347 = Build Array(w504, w502) -> (w501:string[][])
          n348 = Build Array (concatenate)(w512, w516, w517, w508, w507, w501, w495) -> (w494:string[][])
        }
        frame #4 {
          # "spare row"
          n349 = global read "ABB global.vi" "Effy Configuration"() -> (w563:T8)
          n350 = global read "ABB global.vi" "Temperature Scaling"() -> (w571:dbl[][])
          n351 = global read "ABB global.vi" "No load run config"() -> (w555:T7)
          n352 = global read "ABB global.vi" "Bearing run config"() -> (w585:T7)
          n353 = global read "ABB global.vi" "Heat run config"() -> (w600:T7)
          n354 = Unbundle By Name(w585) -> ("category"=w586:i32[], "Category names"=w577:string[], "Category none names"=w576:string[])
          n355 = Unbundle By Name(w555) -> ("category"=w551:i32[], "Category names"=w550:string[], "Category none names"=w547:string[])
          n356 = Unbundle By Name(w563) -> ("Number of Loads"=w562:i32, "Loads (%Rated)"=w561:dbl[])
          n357 = Unbundle By Name(w600) -> ("Category names"=w597:string[], "Category none names"=w594:string[])
          n358 = Number To Fractional String(number=w571, precision (6)=i16 6) -> (F-format string=w565:string[][])  [unwired: 2 in]
          n359 = Array Size(array=w586) -> (size(s)=w587:i32)
          n360 = Array Size(array=w576) -> (size(s)=w579:i32)
          n361 = Array Size(array=w577) -> (size(s)=w580:i32)
          n362 = Array Size(array=w565) -> (size(s)=w569:i32[])
          n363 = Array Size(array=w550) -> (size(s)=w543:i32)
          n364 = Number To Decimal String(number=w587) -> (decimal integer string=w583:string)  [unwired: 1 in]
          n365 = Build Array("No load categories", "3" ("element")) -> (w549:string[])
          n366 = Number To Decimal String(number=w579) -> (decimal integer string=w578:string)  [unwired: 1 in]
          n367 = Number To Decimal String(number=w580) -> (decimal integer string=w581:string)  [unwired: 1 in]
          n368 = Array Size(array=w597) -> (size(s)=w599:i32)
          n369 = Build Array (concatenate)(w562, w561) -> (w560:dbl[])
          n370 = Array Size(array=w594) -> (size(s)=w595:i32)
          n371 = Number To Decimal String(number=w569) -> (decimal integer string=w568:string[])  [unwired: 1 in]
          n372 = Build Array("Heat run Temp categories", "2" ("element")) -> (w592:string[])
          n373 = Array Size(array=w547) -> (size(s)=w546:i32)
          n374 = Number To Decimal String(number=w543) -> (decimal integer string=w542:string)  [unwired: 1 in]
          n375 = Array Size(array=w551) -> (size(s)=w552:i32)
          n376 = Number To Decimal String(number=w586) -> (decimal integer string=w582:string[])  [unwired: 1 in]
          n377 = Number To Decimal String(number=w599) -> (decimal integer string=w598:string)  [unwired: 1 in]
          n378 = Number To Decimal String(number=w595) -> (decimal integer string=w596:string)  [unwired: 1 in]
          n379 = Number To Decimal String(number=w546) -> (decimal integer string=w545:string)  [unwired: 1 in]
          n380 = Build Array (concatenate)(w542, w550) -> (w539:string[])
          n381 = Build Array (concatenate)(w552, w551) -> (w541:i32[])
          n382 = Build Array (concatenate)("Temperature scaling", w568) -> (w566:string[])
          n383 = Build Array("Bearing temp alloc2", "3" ("element")) -> (w575:string[])
          n384 = Number To Fractional String(number=w560, precision (6)=i16 1) -> (F-format string=w558:string[])  [unwired: 2 in]
          n385 = Build Array (concatenate)(w583, w582) -> (w574:string[])
          n386 = Build Array (concatenate)(w578, w576) -> (w572:string[])
          n387 = Build Array (concatenate)(w581, w577) -> (w573:string[])
          n388 = Build Array (concatenate)(w545, w547) -> (w540:string[])
          n389 = Build Array (concatenate)(w596, w594) -> (w590:string[])
          n390 = Build Array (concatenate)(w598, w597) -> (w591:string[])
          n391 = Build Array (concatenate)(w566, w565) -> (w564:string[][])
          n392 = Number To Decimal String(number=w541) -> (decimal integer string=w548:string[])  [unwired: 1 in]
          n393 = Build Array("") -> (w537:string[])
          n394 = Build Array (concatenate)("Efficiencies", w558) -> (w557:string[])
          n395 = Build Array(w549, w548, w539, w540) -> (w544:string[][])
          n396 = global read "ABB global.vi" "VT and CT Ratios"() -> (w536:T9)
          n397 = Unbundle By Name(w536) -> ("VT Primary"=w535:dbl, "VT Secondary"=w534:dbl, "CT  Primary"=w533:dbl, "CT Secondary"=w532:dbl, "Current Shunt"=w531:enum16{"Internal", "External"}, "Averaging interval"=w525:dbl)
          n398 = Build Array(w535, w534, w533, w532, w531, w525) -> (w530:dbl[])
          n399 = Number To Fractional String(number=w530, precision (6)=i16 2) -> (F-format string=w527:string[])  [unwired: 2 in]
          n400 = Build Array (concatenate)("VT&CT ratios", w527) -> (w528:string[])
          n401 = Build Array (concatenate)(w592, w591, w590, w575, w574, w573, w572, w564, w557, w544, w528) -> (w589:string[][])
          n402 = Build Array (concatenate)(w602, w537, w589) -> (w524:string[][])
        }
        frame #5 {
          n403 = global read "ABB global.vi" "Temperature sensors"() -> (w606:string[])
          n404 = while {
            shift-right: [w616] -> _
            shift-left: w606 -> [w622]
            tunnel: [w617] -> w611 mode=indexing
            stop <- w614 stop-if-true
            n405 = Delete From Array(array=w622, length=8, index=0) -> (deleted portion=w618:string[], array with subset deleted=w616:string[])
            n406 = Array Size(array=w618) -> (size(s)=w620:i32)
            n407 = Number To Decimal String(number=w620) -> (decimal integer string=w619:string)  [unwired: 1 in]
            n408 = Array Size(array=w616) -> (size(s)=w615:i32)
            n409 = Build Array (concatenate)(w619, w618) -> (w617:string[])
            n410 = Equal To 0?(x=w615) -> (x = 0?=w614:bool)
          }
          n411 = Array Size(array=w611) -> (size(s)=w607:i32[])
          n412 = Number To Decimal String(number=w607) -> (decimal integer string=w609:string[])  [unwired: 1 in]
          n413 = Build Array (concatenate)("Temp sens", w609) -> (w610:string[])
          n414 = Build Array (concatenate)(w610, w611) -> (w605:string[][])
          n415 = Build Array (concatenate)(w612, w605) -> (w603:string[][])
          n416 = call "ABB Write to spreadsheet.vi"("2D data"=w603, "file path (dialog if empty)"=w604) -> ()  [unwired: 6 in, 1 out]
        }
      }
    }
  }
